vi "Length.vi"(10 "Point 2":T1 {"Y" format="%.2f"; "X" format="%.2f"}, 11 "Point":T1 {"Y" format="%.2f"; "X" format="%.2f"}) -> (3 "Length":sgl)   [LabVIEW 2015]
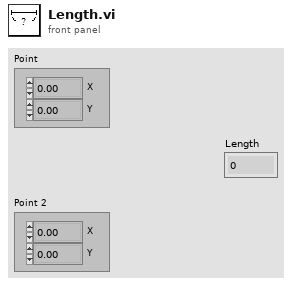
[diagram p1: front panel]
types:
  T1 = typedef "IMAQ Point" = cluster{"X":sgl, "Y":sgl}
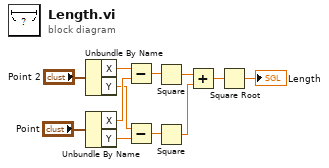
[diagram p0: block diagram]
diagram:
  n1 = Unbundle By Name("Point 2") -> ("X"=w10:sgl, "Y"=w8:sgl)
  n2 = Unbundle By Name("Point") -> ("X"=w9:sgl, "Y"=w7:sgl)
  n3 = Subtract(x=w10, y=w9) -> (x-y=w6:sgl)
  n4 = Subtract(x=w8, y=w7) -> (x-y=w5:sgl)
  n5 = Square(x=w6) -> (x^2=w3:sgl)
  n6 = Square(x=w5) -> (x^2=w4:sgl)
  n7 = Add(x=w3, y=w4) -> (x+y=w2:sgl)
  n8 = Square Root(x=w2) -> (sqrt(x)=→"Length":sgl)
